vi "Asynchronous Read ARINC Words.vi"() -> ()   [LabVIEW 8.6]
uses:
  <libdir>/resource/objmgr/ueidaq.rc
  vi.lib/UeiDaq/UeiDaqCreateARINCInputSession.vi
panel:
  in  "Bits per second":i32(ring) items=["12500", "100000"]
  out "Received Words":i32(listbox)
  out "return count":i32
  out "device name":string
  in  "Resource":string
  out "Total words received":i32
  in  "ARINC words Watermark":i32
  in  "stop":bool
  # "ASYNCHRONOUS READ FROM ARINC-429 PORT"
  # "1/ Set the resource name"
  # "Device info"
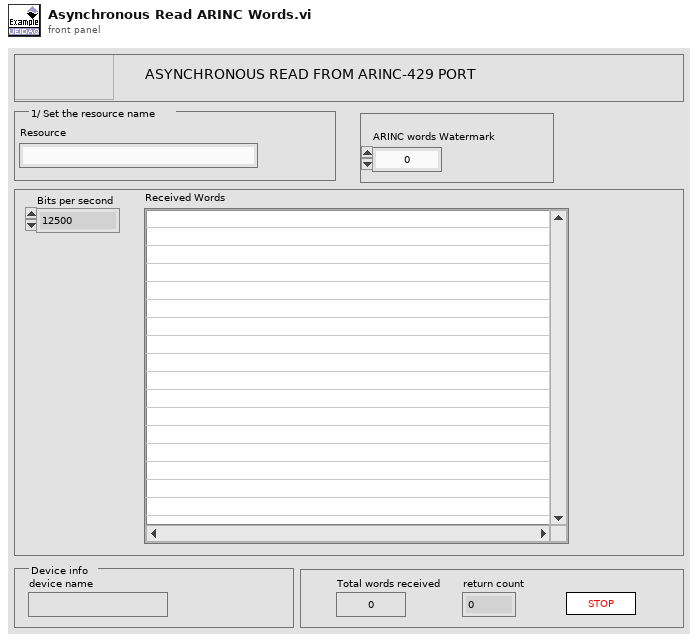
[diagram p1: front panel]
types:
  T1 = cluster{"Label":u16, "Data":u32, "Sdi":u8, "Ssm":u8, "Parity":u8, "Timestamp":dbl}[]
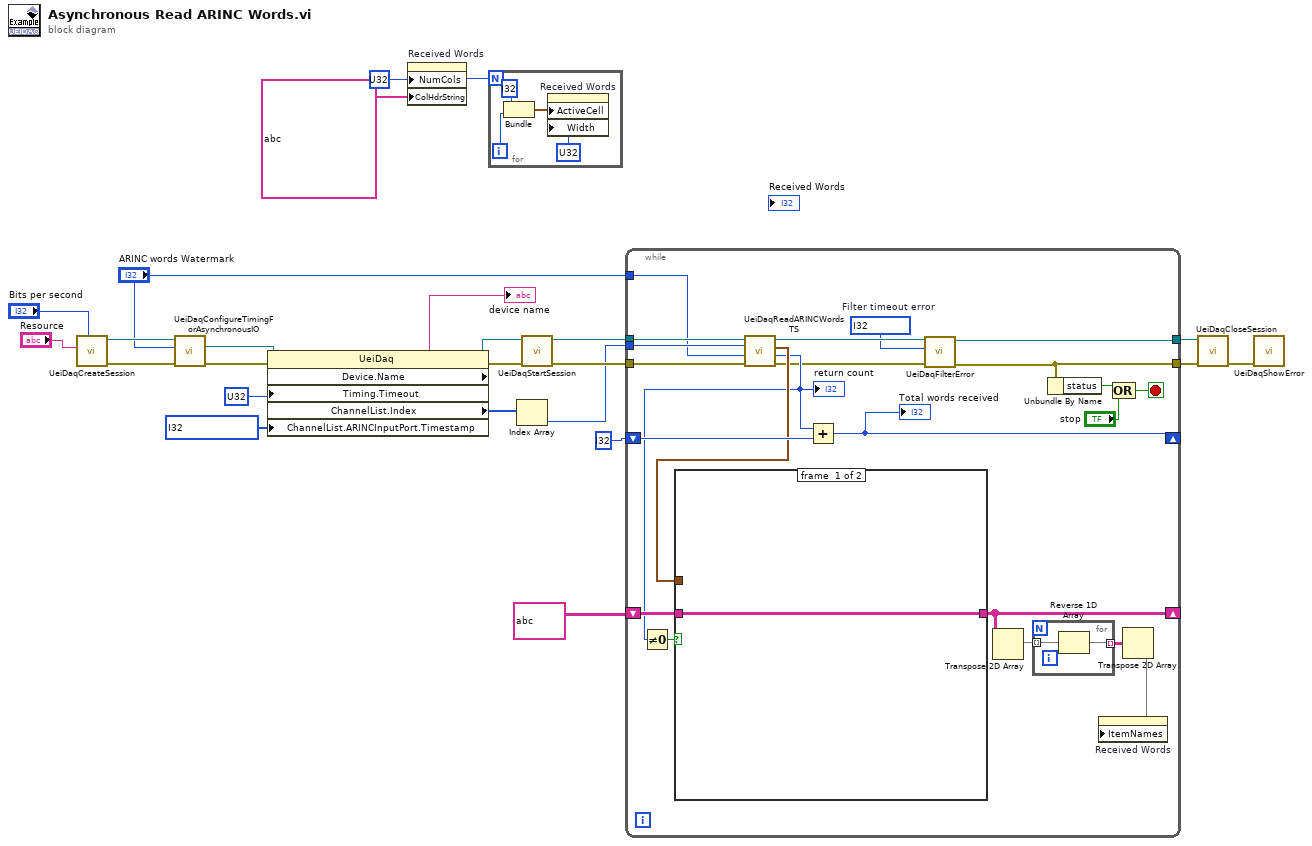
[diagram p0: block diagram]
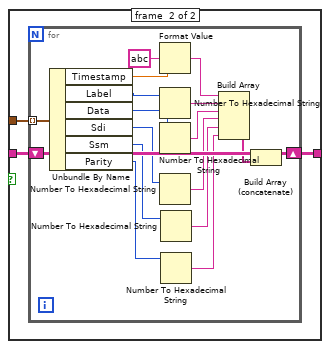
[diagram p2: hidden frame]
diagram:
  w2 = i32[] ? items=["Disable", "Enable"] ("Channel List:ARINC Input Port:Timestamp")
  w10 = u32 ? ("Num Columns")
  n1 = call-poly "UeiDaqCreateSession.vi"("Bits per second"="Bits per second", "Resource"="Resource") -> ("error out"=w21:errorcluster, "UeiDaq Refnum Out"=w22:refnum<k20>)  [unwired: 5 in, 3 out]
  n2 = call "UeiDaqConfigureTimingForAsynchronousIO.vi"("error in (no error)"=w21, "Watermark"="ARINC words Watermark", "UeiDaq Refnum In"=w22) -> ("error out"=w18:errorcluster, "UeiDaq Refnum Out"=w19:refnum<k20>)  [unwired: 7 in]
  n3 = property class="UeiDaq"(reference=w19, error in=w18, "Timing.Timeout"=u32 ? ("Timing:Timeout"), "ChannelList.ARINCInputPort.Timestamp"=w2) -> (reference out=w6:refnum<k20>, error out=w8:errorcluster, "Device.Name"=→"device name":string, "ChannelList.Index"=w4:i32[])
  n4 = property on="Received Words" class="MCListbox (strict)"("NumCols"=w10, "ColHdrString"=string[] ?) -> ()  [unwired: 2 in, 2 out]
  n5 = for {
    N: w10 -> [_]
    i -> [w26]
    n6 = Bundle(i32 ?, w26) -> (w24:cluster{i32, i32})  [unwired: 1 out]
    n7 = property on="Received Words" class="MCListbox (strict)"("ActiveCell"=w24, "Width"=u32 ? ("Cell Size:Width")) -> ()  [unwired: 2 in, 2 out]
  }
  n8 = Index Array(array=w4) -> (element=w3:i32)  [unwired: 1 in]
  n9 = call "UeiDaqStartSession.vi"("error in (no error)"=w8, "UeiDaq Refnum In"=w6) -> ("error out"=w7:errorcluster, "UeiDaq Refnum Out"=w5:refnum<k20>)  [unwired: 8 in]
  n10 = while {
    tunnel: w5 -> [w48]
    tunnel: w7 -> [w49]
    tunnel: [w31] -> w17
    tunnel: [w33] -> w16
    shift-right: [w44] -> _
    shift-left: i32 ? -> [w45]
    shift-right: [w37] -> _
    shift-left: string[][] ? ("Item Names") -> [w42]
    tunnel: w3 -> [w29]
    tunnel: "ARINC words Watermark" -> [w28]
    stop <- w46 stop-if-true
    w30 = i32 ?  # Filter timeout error
    n11 = call "UeiDaqReadARINCWordsTS.vi"("error in (no error)"=w49, "ARINC words count"=w28, "Port"=w29, "UeiDaq Refnum In"=w48) -> ("error out"=w32:errorcluster, "return count"=w40:i32, "Frames"=w43:T1, "UeiDaq Refnum Out"=w34:refnum<k20>)  [unwired: 4 in]
    "return count" <- w40
    n12 = Not Equal To 0?(x=w40) -> (x != 0?=w41:bool)
    n13 = case shown="True" w41 {
      tunnel: w43 -> [_ w55]
      tunnel: w42 -> [w52 w54]
      tunnel: [w52 w53] -> w37
      frame #0 {
      }
      frame #1 {
        n14 = for {
          tunnel: w55 -> [w72] mode=indexing
          shift-right: [w63] -> w53
          shift-left: w54 -> [w71]
          n15 = Unbundle By Name(w72) -> ("Timestamp"=w58:dbl, "Label"=w70:u16, "Data"=w68:u32, "Sdi"=w67:u8, "Ssm"=w62:u8, "Parity"=w61:u8)
          n16 = Format Value(format string=string ?, value (0)=w58) -> (output string=w56:string)  [unwired: 1 in]
          n17 = Number To Hexadecimal String(2:w70) -> (0:w69:string)  [unwired: 1 out]
          n18 = Number To Hexadecimal String(2:w68) -> (0:w66:string)  [unwired: 1 out]
          n19 = Number To Hexadecimal String(2:w67) -> (0:w65:string)  [unwired: 1 out]
          n20 = Number To Hexadecimal String(2:w62) -> (0:w60:string)  [unwired: 1 out]
          n21 = Number To Hexadecimal String(2:w61) -> (0:w59:string)  [unwired: 1 out]
          n22 = Build Array(w56, w69, w66, w65, w60, w59) -> (w64:string[])
          n23 = Build Array (concatenate)(w71, w64) -> (w63:string[][])
        }
      }
    }
    n24 = Add(x=w40, y=w45) -> (x+y=w44:i32)
    "Total words received" <- w44
    n25 = call "UeiDaqFilterError.vi"("error in (no error)"=w32, "Error to filter"=w30, "UeiDaq Refnum In"=w34) -> ("error out"=w31:errorcluster, "UeiDaq Refnum Out"=w33:refnum<k20>)  [unwired: 7 out]
    n26 = Transpose 2D Array(2D array=w37) -> (transposed array=w36:string[][])
    n27 = for {
      tunnel: w36 -> [w51] mode=indexing
      tunnel: [w50] -> w39 mode=indexing
      n28 = Reverse 1D Array(array=w51) -> (reversed array=w50:string[])
    }
    n29 = Unbundle By Name(w31) -> ("status"=w35:bool)
    n30 = Compound Arithmetic op=OR(w35, "stop") -> (w46:bool)
    n31 = Transpose 2D Array(2D array=w39) -> (transposed array=w38:string[][])
    n32 = property on="Received Words" class="MCListbox (strict)"("ItemNames"=w38) -> ()  [unwired: 2 in, 2 out]
  }
  n33 = call "UeiDaqCloseSession.vi"("error in (no error)"=w17, "UeiDaq Refnum In"=w16) -> ("error out"=w23:errorcluster)  [unwired: 1 in, 8 out]
  n34 = call "UeiDaqShowError.vi"("error in (no error)"=w23) -> ()  [unwired: 2 in, 9 out]
